vi "TestACS712.vi"() -> ()   [LabVIEW 2020]
panel:
  out "Waveform Chart":dynamicdata(graph)
  in  "?":bool
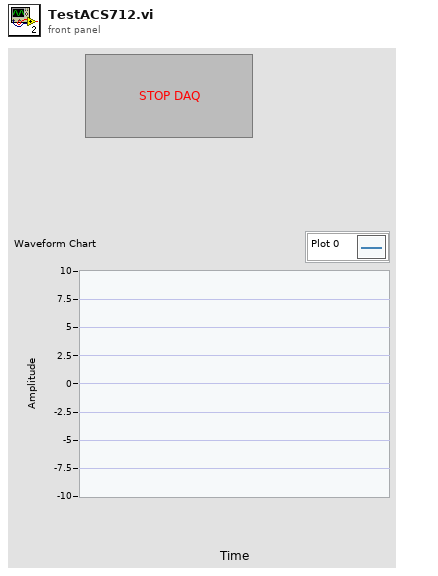
[diagram p1: front panel]
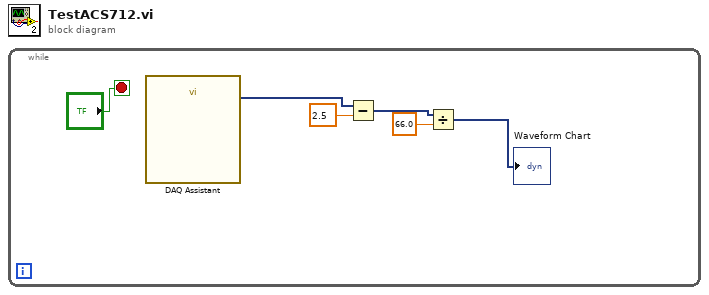
[diagram p0: block diagram]
diagram:
  n1 = while {
    stop <- "?" stop-if-true
    n2 = call "DAQ Assistant"() -> ("data"=w4:dynamicdata)  [unwired: 16 in, 3 out]
    n3 = Subtract(x=w4, y=2.5) -> (x-y=w3:dynamicdata)
    n4 = Divide(x=w3, y=66.0) -> (x/y=→"Waveform Chart":dynamicdata)
  }
